vi "649SetFinal.vi"(0 "?":bool) -> (3 "?":string[][](array[string]))   [LabVIEW 2023]
uses:
  <vilib>/numeric/Random Number (Range) U64.vi
  <vilib>/numeric/sub_Random U32.vi
  <vilib>/Utility/file.llb/Write Delimited Spreadsheet (string).vi
panel:
  out "error out 2":errorcluster
  out "error out":errorcluster
  out "?":string[](array[string])
  # "6@49"
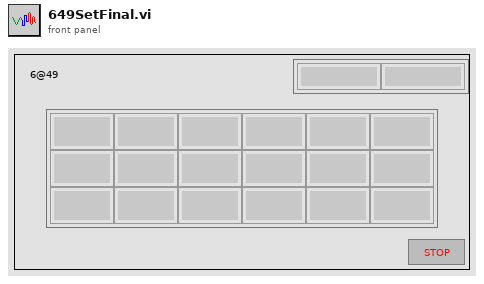
[diagram p1: front panel]
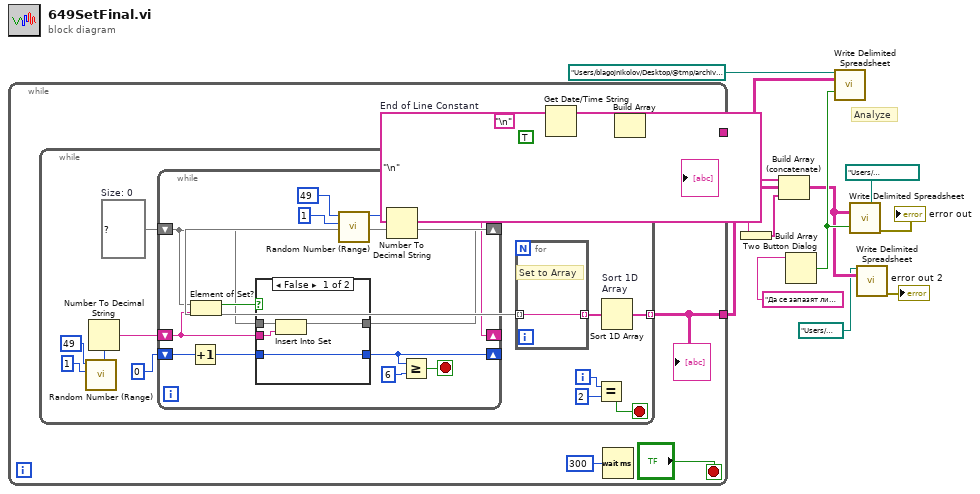
[diagram p0: block diagram]
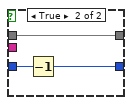
[diagram p2: hidden frame]
diagram:
  w9 = "\n"  # End of Line Constant
  # "Analyze"
  n1 = while {
    tunnel: [w20] -> w8
    tunnel: [w14] -> w12
    stop <- "?" stop-if-true
    n2 = while {
      tunnel: [w21] -> w20 mode=indexing
      i -> [w27]
      stop <- w25 stop-if-true
      w32 = set{string} {}  # Size: 0
      n3 = call-poly <vilib>:"Random Number (Range).vi"("lower bound (0)"=u64 1, "upper bound (100)"=u64 49) -> ("number"=w29:u64)  [unwired: 9 in]
      n4 = Number To Decimal String(number=w29) -> (decimal integer string=w28:string)  [unwired: 1 in]
      n5 = while {
        shift-right: [w37] -> _
        shift-left: w28 -> [w38]
        shift-right: [w44] -> w23
        shift-left: w32 -> [w45]
        shift-right: [w36] -> _
        shift-left: 0 -> [w35]
        stop <- w43 stop-if-true
        n6 = Increment(x=w35) -> (x+1=w34:i32)
        n7 = Element of Set?(10:w38, 11:w45) -> (3:w46:bool)
        n8 = case shown="False" w46 {
          tunnel: w45 -> [w50 w53]
          tunnel: [w49 w53] -> w44
          tunnel: w34 -> [w48 w52]
          tunnel: [w48 w51] -> w36
          tunnel: w38 -> [w47 _]
          frame False {
            n9 = Insert Into Set(10:w47, 11:w50) -> (3:w49:set{string})  [unwired: 1 out]
          }
          frame True {
            n10 = Decrement(x=w52) -> (x-1=w51:i32)
          }
        }
        n11 = call-poly <vilib>:"Random Number (Range).vi"("lower bound (0)"=u64 1, "upper bound (100)"=u64 49) -> ("number"=w39:u64)  [unwired: 9 in]
        n12 = Number To Decimal String(number=w39) -> (decimal integer string=w37:string)  [unwired: 1 in]
        n13 = Greater Or Equal?(x=w36, y=6) -> (x >= y?=w43:bool)
      }
      n14 = for {
        tunnel: [w33] -> w22 mode=indexing
        tunnel: w23 -> [w33] mode=indexing
        # "Set to Array"
      }
      n15 = Equal?(x=w27, y=2) -> (x = y?=w25:bool)
      n16 = Sort 1D Array "Sort 1D \nArray"(array=w22) -> (sorted array=w21:string[])
    }
    "?" <- w20
    n17 = Get Date/Time String(want seconds? (F)=TRUE) -> (date string=w16:string, time string=w17:string)  [unwired: 2 in]
    n18 = Wait (ms)(milliseconds to wait=u32 300) -> ()  [unwired: 1 out]
    n19 = Build Array(w16, w17, "\n") -> (w14:string[])
    "?" <- w14
  }
  n20 = Build Array(w9) -> (w11:string[])
  n21 = Build Array (concatenate) "Build Array"(w12, w8, w11) -> (w3:string[][])
  n22 = Two Button Dialog(message="Да се запазят ли предишните резултати ?") -> (T button?=w5:bool)  [unwired: 2 in]
  n23 = call-poly <vilib>:"Write Delimited Spreadsheet.vi"("file path (dialog if empty)"=path "/Users/blagojnikolov/Desktop/@tmp/archive.txt", "2D data"=w8, "append to file? (new file:F)"=w5) -> ()  [unwired: 11 in, 2 out]
  n24 = call-poly <vilib>:"Write Delimited Spreadsheet.vi"("file path (dialog if empty)"=path "/Users/blagojnikolov/Desktop/@tmp/toto.txt", "2D data"=w3, "append to file? (new file:F)"=w5) -> ("error out"=→"error out":errorcluster)  [unwired: 11 in, 1 out]
  n25 = call-poly <vilib>:"Write Delimited Spreadsheet.vi"("file path (dialog if empty)"=path "/Users/blagojnikolov/Desktop/@tmp/checkRes.txt", "2D data"=w3) -> ("error out"=→"error out 2":errorcluster)  [unwired: 12 in, 1 out]
